vi "Destroy_DVR.vi"(8 "error in (no error)":errorcluster, 11 "EVE reference":refnum<data-value>) -> (0 "error out":errorcluster, 3 "EVE out":refnum<class "EVE.lvclass">)   [LabVIEW 2013, in "EVE.lvclass"]
uses:
  EVE.lvclass
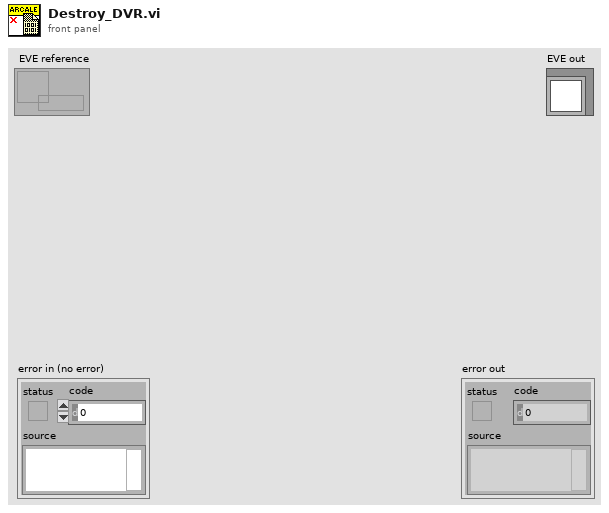
[diagram p1: front panel]
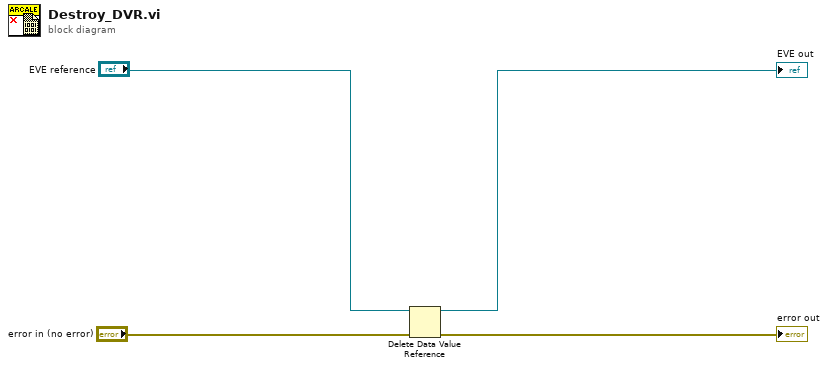
[diagram p0: block diagram]
diagram:
  n1 = Delete Data Value Reference(data value reference="EVE reference", error in="error in (no error)") -> (data value=→"EVE out":refnum<class "EVE.lvclass">, error out=→"error out":errorcluster)
